vi "PH_StatusHandler.set Status.vi"(1 "Service ID Status":i32=-1, 2 "Ring in":refnum<vi>, 3 "Status":T1 items=["no info", "off/false/out", "on/true/in", "Failure", "Alarm", "Status 1", "Status 2", "Status 3"], 4 "Blinking (false)":bool, 5 "error in (no error)":errorcluster, 7 "Tip Strip":string="N/A") -> (19 "error out":errorcluster)   [LabVIEW 2014, in "PH_StatusHandler.lvlib"]
doc: "This VI sets the connected GUI element and updates the DIM service."
uses:
  PH_StatusHandler.lvlib
  PH_StatusHandler.Status.ctl
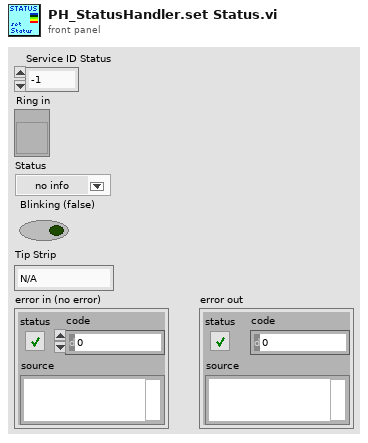
[diagram p1: front panel]
types:
  T1 = typedef "PH_StatusHandler.lvlib/PH_StatusHandler.Status.ctl" = i16
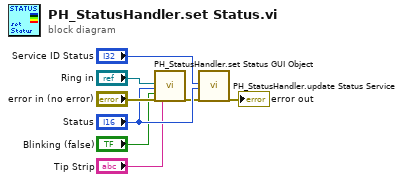
[diagram p0: block diagram]
diagram:
  n1 = call "PH_StatusHandler.set Status GUI Object.vi"("PH Status Ref"="Ring in", "Value"="Status", "Blinking (false)"="Blinking (false)", "error in (no error)"="error in (no error)", "Tip Strip"="Tip Strip") -> ("error out"=w5:errorcluster)  [unwired: 14 in]
  n2 = call "PH_StatusHandler.update Status Service.vi"("Service ID"="Service ID Status", "Status"="Status", "error in (no error)"=w5) -> ("error out"=→"error out":errorcluster)  [unwired: 16 in]
